vi "tsdiag_can_routine_control_1.vi"(6 "data in":u8[](array[numeric]) format="%.0x", 7 "mode":u8(ring)=1 items=["Start routine"=1, "Stop routine"=2, "Request routine results"=3], 8 "error in (no error)":errorcluster, 9 "ID":u16 format="%.0x", 10 "ADiagModuleIndex":i32, 11 "path":path) -> (0 "error out":errorcluster, 1 "success?":bool, 2 "Return Type":i32, 3 "path out":path, 4 "data out":u8[](array[numeric]) format="%.0x")   [LabVIEW 2014]
doc: "31服务，例程控制。"
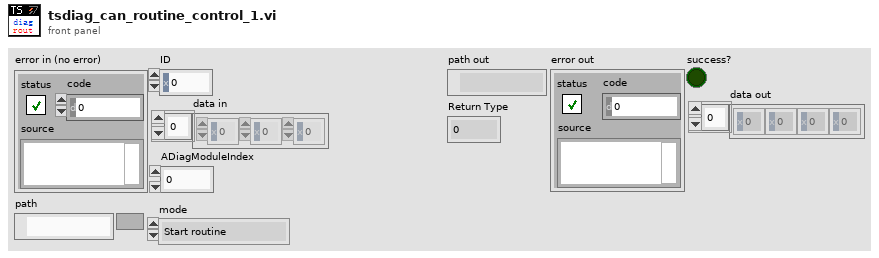
[diagram p1: front panel]
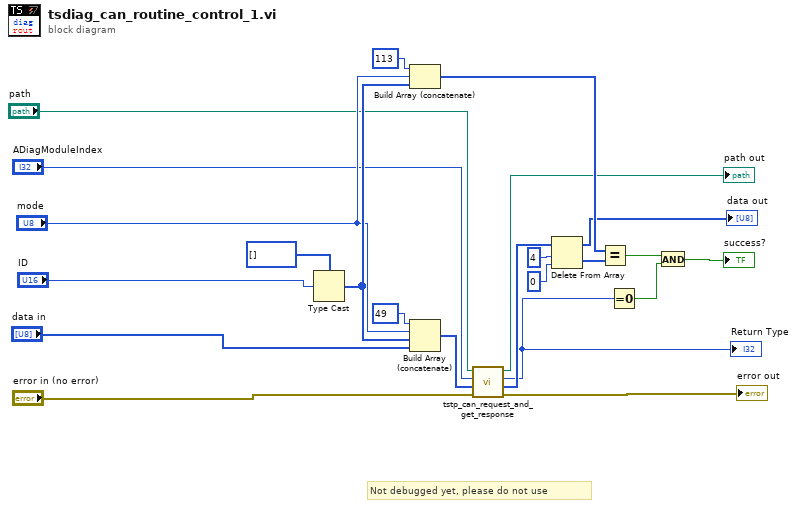
[diagram p0: block diagram]
diagram:
  # "Not debugged yet, please do not use"
  n1 = Type Cast(type=u8[] [], x="ID") -> (*(type *) &x=w14:u8[])
  n2 = Build Array (concatenate)(u8 113 ("element"), "mode", w14) -> (w21:u8[])
  n3 = Build Array (concatenate)(u8 49 ("element"), "mode", w14, "data in") -> (w6:u8[])
  n4 = call "tstp_can_request_and_get_response.vi"("错误输入（无错误）"="error in (no error)", "AReqDataArray"=w6, "ADiagModuleIndex"="ADiagModuleIndex", "path"="path") -> ("错误输出"=→"error out":errorcluster, "Diagnostic response"=w3:u8[], "Return Type"=w2:i32, "path out"=→"path out":path)  [unwired: 4 in]
  "Return Type" <- w2
  n5 = Delete From Array(array=w3, length=4, index=0) -> (deleted portion=w20:u8[], array with subset deleted=→"data out":u8[])
  n6 = Equal?(x=w21, y=w20) -> (x = y?=w18:bool)
  n7 = Equal To 0?(x=w2) -> (x = 0?=w1:bool)
  n8 = And(x=w18, y=w1) -> (x .and. y?=→"success?":bool)
